vi "Read Table Control.vi"(8 "error in (no error)":errorcluster, 11 "Geocoding in":refnum<class "Geocoding.lvclass">) -> (0 "error out":errorcluster, 2 "Table Control":refnum<vi>, 3 "Geocoding out":refnum<class "Geocoding.lvclass">)   [LabVIEW 2025, in "Geocoding Actor.lvlib" / "Geocoding.lvclass"]
uses:
  Geocoding.lvclass
  Geocoding.lvclass/Geocoding.ctl
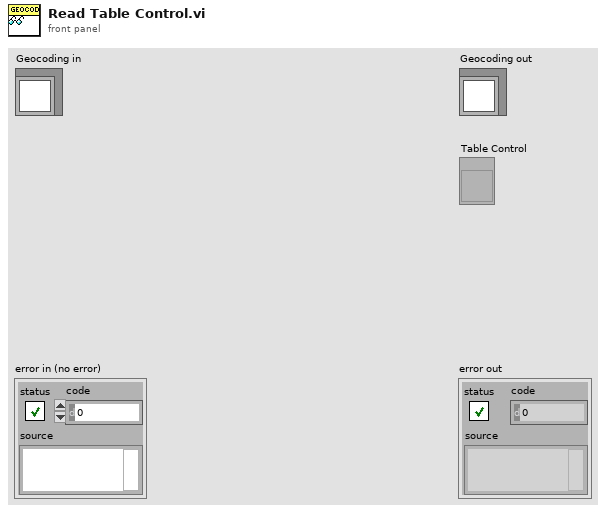
[diagram p1: front panel]
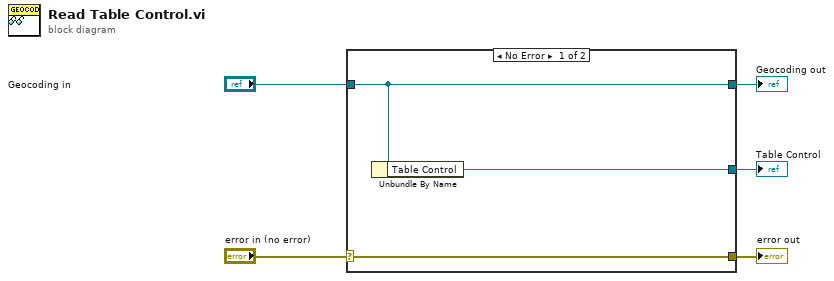
[diagram p0: block diagram]
diagram:
  n1 = case shown="No Error" "error in (no error)" {
    selector: "error in (no error)" -> [w8 w9]
    tunnel: [w8 w9] -> w4
    tunnel: [w7 w10] -> w2
    tunnel: "Geocoding in" -> [w7 w10]
    tunnel: [w6 _] -> w1
    frame No Error {
      n2 = Unbundle By Name(w7) -> ("Table Control"=w6:refnum<vi>)
    }
    frame Error {
    }
  }
  "error out" <- w4
  "Geocoding out" <- w2
  "Table Control" <- w1
